vi "Construct - File.vi"(10 "section":string, 11 "config file":path) -> (0 "Error Out":errorcluster, 3 "Text File":refnum<class "Text File.lvclass">)   [LabVIEW 2019, in "TSC Event Logger.lvlib" / "Text File.lvclass"]
uses:
  Text File.lvclass
  C:/Development/Reuse-libraries/Event Logger/Log Sinks/Log Sinks.lvclass
  Text File.lvclass/Text File.ctl
  <vilib>/Utility/config.llb/Read Key (Path).vi
  <vilib>/Utility/config.llb/Read Key (String).vi
  <vilib>/Utility/config.llb/Read Key (Double).vi
  <vilib>/Utility/config.llb/Read Key (U32).vi
  <vilib>/Utility/config.llb/NI_LVConfig.lvlib
  Log Sinks.lvclass
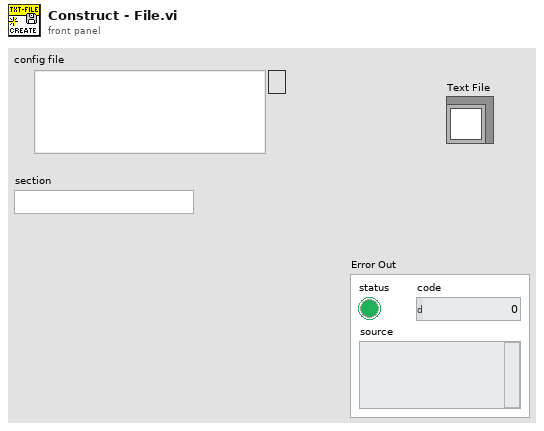
[diagram p1: front panel]
types:
  T1 = typedef "NI_LVConfig.lvlib/Config Data RefNum.ctl" = refnum<k1>
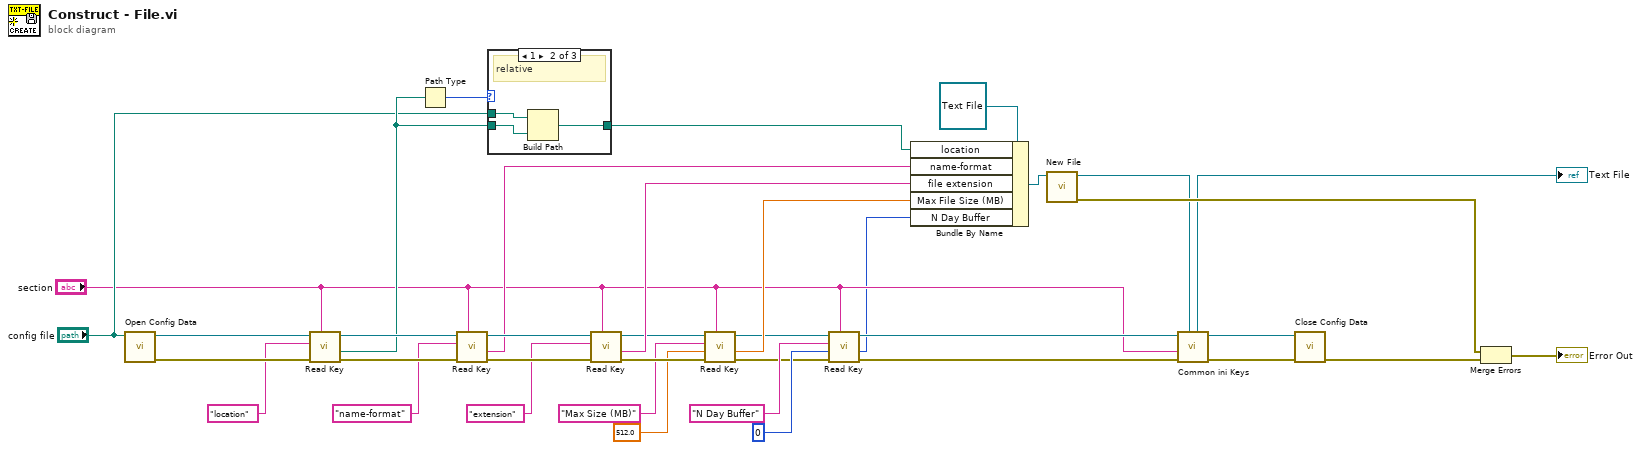
[diagram p0: block diagram]
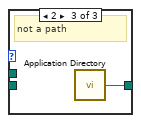
[diagram p3: hidden frame]
diagram:
  n1 = call <vilib>:"Open Config Data.vi"("configuration file path"="config file") -> ("error out"=w36:errorcluster, "refnum"=w34:T1)  [unwired: 8 in, 1 out]
  n2 = call-poly <vilib>:"Read Key.vi"("section"="section", "error in (no error)"=w36, "key"="location", "refnum"=w34) -> ("error out"=w35:errorcluster, "value"=w11:path, "refnum out"=w31:T1)  [unwired: 4 in, 1 out]
  n3 = Path Type(1:w11) -> (0:w12:i16)
  n4 = call-poly <vilib>:"Read Key.vi"("section"="section", "error in (no error)"=w35, "key"="name-format", "refnum"=w31) -> ("error out"=w32:errorcluster, "value"=w23:string, "refnum out"=w28:T1)  [unwired: 4 in, 1 out]
  n5 = case shown="1" w12 {
    tunnel: w11 -> [w38 w40 _]
    tunnel: [w38 w39 w42] -> w10
    tunnel: "config file" -> [_ w41 _]
    frame 0, Default {
      # "absolute"
    }
    frame 1 {
      # "relative"
      n6 = Build Path(base path=w41, name or relative path=w40) -> (appended path=w39:path)
    }
    frame 2 {
      # "not a path"
      n7 = call <vilib>:"Application Directory.vi"() -> ("Application Directory"=w42:path)
    }
  }
  n8 = call-poly <vilib>:"Read Key.vi"("section"="section", "error in (no error)"=w32, "key"="extension", "refnum"=w28) -> ("error out"=w29:errorcluster, "value"=w21:string, "refnum out"=w20:T1)  [unwired: 4 in, 1 out]
  n9 = call-poly <vilib>:"Read Key.vi"("section"="section", "error in (no error)"=w29, "default value"=512.0, "key"="Max Size (MB)", "refnum"=w20) -> ("error out"=w6:errorcluster, "value"=w17:dbl, "refnum out"=w5:T1)  [unwired: 3 in, 1 out]
  n10 = call-poly <vilib>:"Read Key.vi"("section"="section", "error in (no error)"=w6, "default value"=u32 0, "key"="N Day Buffer", "refnum"=w5) -> ("error out"=w4:errorcluster, "value"=w1:u32, "refnum out"=w3:T1)  [unwired: 3 in, 1 out]
  n11 = Bundle By Name(cluster=refnum<class "Text File.lvclass"> refnum ("TSC Event Logger.lvlib:Text File.lvclass"), "location"=w10, "name-format"=w23, "file extension"=w21, "Max File Size (MB)"=w17, "N Day Buffer"=w1) -> (w22:refnum<class "Text File.lvclass">)
  n12 = call "New File.vi"("Text File in"=w22) -> ("error out"=w25:errorcluster, "Text File out"=w15:refnum<class "Text File.lvclass">)  [unwired: 9 in]
  n13 = call "Common ini Keys.vi"("Log Sinks in"=w15, "error in (no error)"=w4, "section"="section", "refnum in"=w3) -> ("error out"=w16:errorcluster, "refnum out"=w13:T1, "Log Sinks out"=→"Text File":refnum<class "Text File.lvclass">)  [unwired: 5 in]
  n14 = call <vilib>:"Close Config Data.vi"("error in (no error)"=w16, "refnum"=w13) -> ("error out"=w37:errorcluster)  [unwired: 8 in, 1 out]
  n15 = Merge Errors(w25, w37) -> (→"Error Out":errorcluster)
